vi "SVT Start Swept Sine (DAQmx).vi"(8 "error in (no error)":errorcluster, 11 "swept sine task in":T1={"source settings"={"AO task name"="", "source"=[]}, "stimulus settings"={"stimulus task name"="", "stimulus"=[]}, "response(s) settings"={"response task name"="", "response"=[]}, "measurement settings"={"AI sampling frequency"=51200.0, "AO sampling frequency"=1024.0, "AI block size"=1024, "AO block Size"=1024, "block duration [ms]"=0.0, "number of AI channels"=0, "device propagation delay [samples]"=0.0, "total propagation time [samples]"=0.0, "DUT propagation time [ms]"=0.0}, "linlog"=enum."linear", "repeat"=enum."off", "frequency list"=[1.0], "amplitude list"=[1.0], "settling time"={"settle time"=0.015599999576807022, "settle cycles"=5}, "integration time"={"integration time"=0.015599999576807022, "integration cycles"=5}, "frequencies indices"={"AI freq index"=0, "AO freq index"=5}, "read marks"={"write index"=0, "read index"=0, "freq start index"=0, "freq stop index"=0, "# extracted"=0, "buffer type"=enum."Invalid buffer", "read/write indices"=[], "AO index"=0, "AI index"=0, "settled"=FALSE, "integration done"=FALSE}, "harmonic settings"={"maximum THD harmonic"=5, "harmonic mapping"=[1], "units"={"THD unit"=enum."%", "nth harmonic unit"=enum."%", "SINAD unit"=enum."dB", "THD+N unit"=enum."dB"}}, "auto resolution settings"={"auto max step"=512, "slow threshold db"=6.0, "fast threshold db"=1.0}, "auto level settings"={"auto level enable"=FALSE, "auto level channel"=6, "ideal ref"=1.0, "max level"=10.0, "ref upper deviation db"=3.0, "ref lower deviation db"=-3.0}, "offset"=1.0, "ramping rate"=0.0, "phase"=1.0, "initialize"=FALSE} {"phase" format="%.2f"; "response(s) settings"."response"."channel info"."pregain" format="%.2f"; "response(s) settings"."response"."channel info"."weighting filter" items=["Linear", "A-weighting", "B-weighting", "C-weighting", "ITU-R 468-4", "Dolby", "CCITT", "C-message", "Wb", "Wc", "Wd", "We", "Wf", "Wh", "Wj", "Wk", "Wm", "AES17 20 kHz lowpass", "AES17 40 kHz lowpass", "AES17 20 kHz highpass", "AES17 40 kHz highpass"]; "response(s) settings"."response"."channel info"."dB reference" format="%^.1e"; "response(s) settings"."response"."channel info"."engineering units" items=["custom..."=0, "V"=1, "A"=21, "C"=30, "pC"=31, "s"=32, "-"=29, "Pa"=2, "N"=20, "g"=3, "m/s^2"=4, "m/s"=5, "m"=6, "mm/s"=12, "mm"=13, "micron/s"=14, "micron"=15, "in/s^2"=7, "in/s"=8, "in"=9, "mil/s"=10, "mil"=11, "rad/s^2"=16, "rad/s"=17, "rad"=18, "deg/s^2"=26, "deg/s"=27, "deg"=28, "RPM"=22, "cycle/s^2"=23, "Hz"=24, "cycle"=25, "strain"=19]; "response(s) settings"."response"."channel info"."sensor sensitivity" format="%#_5f"; "stimulus settings"."stimulus"."channel info"."pregain" format="%.2f"; "stimulus settings"."stimulus"."channel info"."weighting filter" items=["Linear", "A-weighting", "B-weighting", "C-weighting", "ITU-R 468-4", "Dolby", "CCITT", "C-message", "Wb", "Wc", "Wd", "We", "Wf", "Wh", "Wj", "Wk", "Wm", "AES17 20 kHz lowpass", "AES17 40 kHz lowpass", "AES17 20 kHz highpass", "AES17 40 kHz highpass"]; "stimulus settings"."stimulus"."channel info"."dB reference" format="%^.1e"; "stimulus settings"."stimulus"."channel info"."engineering units" items=["custom..."=0, "V"=1, "A"=21, "C"=30, "pC"=31, "s"=32, "-"=29, "Pa"=2, "N"=20, "g"=3, "m/s^2"=4, "m/s"=5, "m"=6, "mm/s"=12, "mm"=13, "micron/s"=14, "micron"=15, "in/s^2"=7, "in/s"=8, "in"=9, "mil/s"=10, "mil"=11, "rad/s^2"=16, "rad/s"=17, "rad"=18, "deg/s^2"=26, "deg/s"=27, "deg"=28, "RPM"=22, "cycle/s^2"=23, "Hz"=24, "cycle"=25, "strain"=19]; "stimulus settings"."stimulus"."channel info"."sensor sensitivity" format="%#_5f"; "ramping rate" format="%.4f"; "offset" format="%.2f"; "auto level settings"."ref lower deviation db" format="%.4f"; "auto level settings"."ref upper deviation db" format="%.4f"; "auto level settings"."max level" format="%.4f"; "auto level settings"."ideal ref" format="%.4f"; "auto resolution settings"."fast threshold db" format="%.4f"; "auto resolution settings"."slow threshold db" format="%.4f"; "harmonic settings"."maximum THD harmonic" max=10 step=1; "integration time"."integration time" format="%.2p"; "settling time"."settle time" format="%.2p"; "amplitude list" format="%.2f"; "frequency list" format="%.2f"; "measurement settings"."DUT propagation time [ms]" format="%.2f"; "measurement settings"."AO sampling frequency" format="%.2f"; "measurement settings"."AI sampling frequency" format="%.2f"}) -> (0 "error out":errorcluster, 3 "swept sine task out":T1={"source settings"={"AO task name"="", "source"=[]}, "stimulus settings"={"stimulus task name"="", "stimulus"=[]}, "response(s) settings"={"response task name"="", "response"=[]}, "measurement settings"={"AI sampling frequency"=51200.0, "AO sampling frequency"=1024.0, "AI block size"=1024, "AO block Size"=1024, "block duration [ms]"=0.0, "number of AI channels"=0, "device propagation delay [samples]"=0.0, "total propagation time [samples]"=0.0, "DUT propagation time [ms]"=0.0}, "linlog"=enum."linear", "repeat"=enum."off", "frequency list"=[1.0], "amplitude list"=[1.0], "settling time"={"settle time"=0.015599999576807022, "settle cycles"=5}, "integration time"={"integration time"=0.015599999576807022, "integration cycles"=5}, "frequencies indices"={"AI freq index"=0, "AO freq index"=5}, "read marks"={"write index"=0, "read index"=0, "freq start index"=0, "freq stop index"=0, "# extracted"=0, "buffer type"=enum."Invalid buffer", "read/write indices"=[], "AO index"=0, "AI index"=0, "settled"=FALSE, "integration done"=FALSE}, "harmonic settings"={"maximum THD harmonic"=5, "harmonic mapping"=[1], "units"={"THD unit"=enum."%", "nth harmonic unit"=enum."%", "SINAD unit"=enum."dB", "THD+N unit"=enum."dB"}}, "auto resolution settings"={"auto max step"=512, "slow threshold db"=6.0, "fast threshold db"=1.0}, "auto level settings"={"auto level enable"=FALSE, "auto level channel"=6, "ideal ref"=1.0, "max level"=10.0, "ref upper deviation db"=3.0, "ref lower deviation db"=-3.0}, "offset"=1.0, "ramping rate"=0.0, "phase"=1.0, "initialize"=FALSE} {"phase" format="%.2f"; "response(s) settings"."response"."channel info"."pregain" format="%.2f"; "response(s) settings"."response"."channel info"."weighting filter" items=["Linear", "A-weighting", "B-weighting", "C-weighting", "ITU-R 468-4", "Dolby", "CCITT", "C-message", "Wb", "Wc", "Wd", "We", "Wf", "Wh", "Wj", "Wk", "Wm", "AES17 20 kHz lowpass", "AES17 40 kHz lowpass", "AES17 20 kHz highpass", "AES17 40 kHz highpass"]; "response(s) settings"."response"."channel info"."dB reference" format="%^.1e"; "response(s) settings"."response"."channel info"."engineering units" items=["custom..."=0, "V"=1, "A"=21, "C"=30, "pC"=31, "s"=32, "-"=29, "Pa"=2, "N"=20, "g"=3, "m/s^2"=4, "m/s"=5, "m"=6, "mm/s"=12, "mm"=13, "micron/s"=14, "micron"=15, "in/s^2"=7, "in/s"=8, "in"=9, "mil/s"=10, "mil"=11, "rad/s^2"=16, "rad/s"=17, "rad"=18, "deg/s^2"=26, "deg/s"=27, "deg"=28, "RPM"=22, "cycle/s^2"=23, "Hz"=24, "cycle"=25, "strain"=19]; "response(s) settings"."response"."channel info"."sensor sensitivity" format="%#_5f"; "stimulus settings"."stimulus"."channel info"."pregain" format="%.2f"; "stimulus settings"."stimulus"."channel info"."weighting filter" items=["Linear", "A-weighting", "B-weighting", "C-weighting", "ITU-R 468-4", "Dolby", "CCITT", "C-message", "Wb", "Wc", "Wd", "We", "Wf", "Wh", "Wj", "Wk", "Wm", "AES17 20 kHz lowpass", "AES17 40 kHz lowpass", "AES17 20 kHz highpass", "AES17 40 kHz highpass"]; "stimulus settings"."stimulus"."channel info"."dB reference" format="%^.1e"; "stimulus settings"."stimulus"."channel info"."engineering units" items=["custom..."=0, "V"=1, "A"=21, "C"=30, "pC"=31, "s"=32, "-"=29, "Pa"=2, "N"=20, "g"=3, "m/s^2"=4, "m/s"=5, "m"=6, "mm/s"=12, "mm"=13, "micron/s"=14, "micron"=15, "in/s^2"=7, "in/s"=8, "in"=9, "mil/s"=10, "mil"=11, "rad/s^2"=16, "rad/s"=17, "rad"=18, "deg/s^2"=26, "deg/s"=27, "deg"=28, "RPM"=22, "cycle/s^2"=23, "Hz"=24, "cycle"=25, "strain"=19]; "stimulus settings"."stimulus"."channel info"."sensor sensitivity" format="%#_5f"; "ramping rate" format="%.4f"; "offset" format="%.2f"; "auto level settings"."ref lower deviation db" format="%.4f"; "auto level settings"."ref upper deviation db" format="%.4f"; "auto level settings"."max level" format="%.4f"; "auto level settings"."ideal ref" format="%.4f"; "auto resolution settings"."fast threshold db" format="%.4f"; "auto resolution settings"."slow threshold db" format="%.4f"; "harmonic settings"."maximum THD harmonic" max=10 step=1; "integration time"."integration time" format="%.2p"; "settling time"."settle time" format="%.2p"; "amplitude list" format="%.2f"; "frequency list" format="%.2f"; "measurement settings"."DUT propagation time [ms]" format="%.2f"; "measurement settings"."AO sampling frequency" format="%.2f"; "measurement settings"."AI sampling frequency" format="%.2f"})   [LabVIEW 2017, in "SoundVib_SweptSine.lvlib"]
doc: "Starts the swept-sine measurement."
uses:
  <vilib>/addons/Sound and Vibration/svt_Swept Sine/SoundVib_SweptSine.lvlib
  <vilib>/addons/Sound and Vibration/svt_Swept Sine/subVIs/sv_Swept Sine Task.ctl
  <vilib>/addons/_NISVFA/_Shared subVIs/Controls/svc_Channel Info.ctl
  <vilib>/addons/_NISVFA/_Shared subVIs/Controls/svc_Engineering Units Text Ring.ctl
  <vilib>/addons/_NISVFA/_Shared subVIs/Controls/svc_Weighting Filter Text Ring.ctl
  <vilib>/DAQmx/write.llb/DAQmx Write (Analog 1D DBL 1Chan NSamp).vi
  <vilib>/DAQmx/miscellaneous.llb/DAQmx Fill In Error Info.vi
  <vilib>/DAQmx/configure/trigger.llb/DAQmx Start Trigger (Digital Edge).vi
  <resource>/objmgr/daqmx.rc
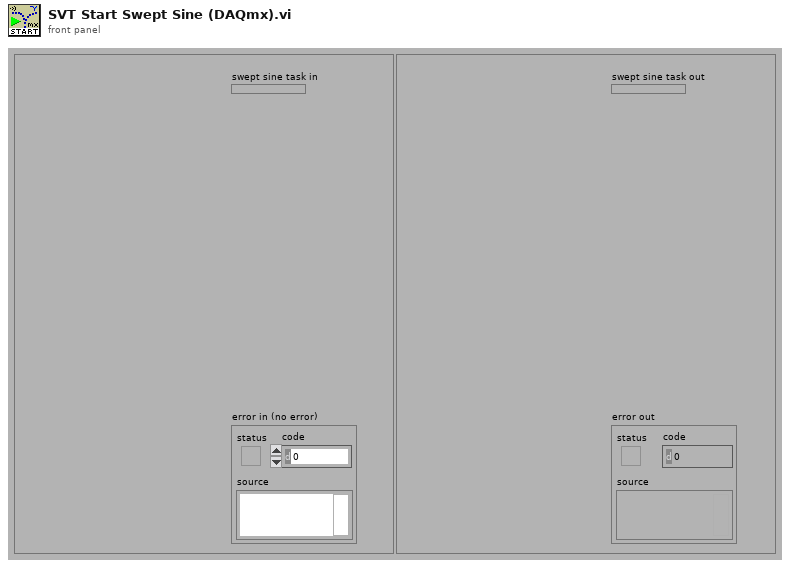
[diagram p1: front panel]
types:
  T1 = typedef "SoundVib_SweptSine.lvlib/sv_Swept Sine Task.ctl" = cluster{"source settings":cluster{"AO task name":refnum<k21>, "source":cluster{"AO physical channel":tag}[]}, "stimulus settings":cluster{"stimulus task name":refnum<k21>, "stimulus":cluster{"stimulus physical channel":tag, "channel info":T2}[]}, "response(s) settings":cluster{"response task name":refnum<k21>, "response":cluster{"response physical channel":tag, "channel info":T2}[]}, "measurement settings":cluster{"AI sampling frequency":dbl, "AO sampling frequency":dbl, "AI block size":i32, "AO block Size":i32, "block duration [ms]":dbl, "number of AI channels":i32, "device propagation delay [samples]":dbl, "total propagation time [samples]":dbl, "DUT propagation time [ms]":dbl}, "linlog":enum16{"linear", "log"}, "repeat":enum16{"off", "on"}, "frequency list":dbl[], "amplitude list":dbl[], "settling time":cluster{"settle time":dbl, "settle cycles":i32}, "integration time":cluster{"integration time":dbl, "integration cycles":i32}, "frequencies indices":cluster{"AI freq index":i32, "AO freq index":i32}, "read marks":cluster{"write index":u32, "read index":u32, "freq start index":u32, "freq stop index":u32, "# extracted":u32, "buffer type":enum16{"Invalid buffer", "Intermediate buffer", "Final buffer"}, "read/write indices":cluster{"settle time index":u32, "integration time index":u32}[], "AO index":i32, "AI index":i32, "settled":bool, "integration done":bool}, "harmonic settings":cluster{"maximum THD harmonic":u32, "harmonic mapping":u32[], "units":cluster{"THD unit":enum16{"dB", "%"}, "nth harmonic unit":enum16{"dB", "%"}, "SINAD unit":enum16{"dB", "%"}, "THD+N unit":enum16{"dB", "%"}}}, "auto resolution settings":cluster{"auto max step":i32, "slow threshold db":dbl, "fast threshold db":dbl}, "auto level settings":cluster{"auto level enable":bool, "auto level channel":u8, "ideal ref":sgl, "max level":sgl, "ref upper deviation db":sgl, "ref lower deviation db":sgl}, "offset":dbl, "ramping rate":dbl, "phase":dbl, "initialize":bool}
  T2 = typedef "svc_Channel Info.ctl" = cluster{"sensor sensitivity":dbl, "engineering units":T3, "dB reference":dbl, "custom label":string, "weighting filter":T4, "pregain":dbl}
  T3 = typedef "svc_Engineering Units Text Ring.ctl" = u16
  T4 = typedef "svc_Weighting Filter Text Ring.ctl" = u16
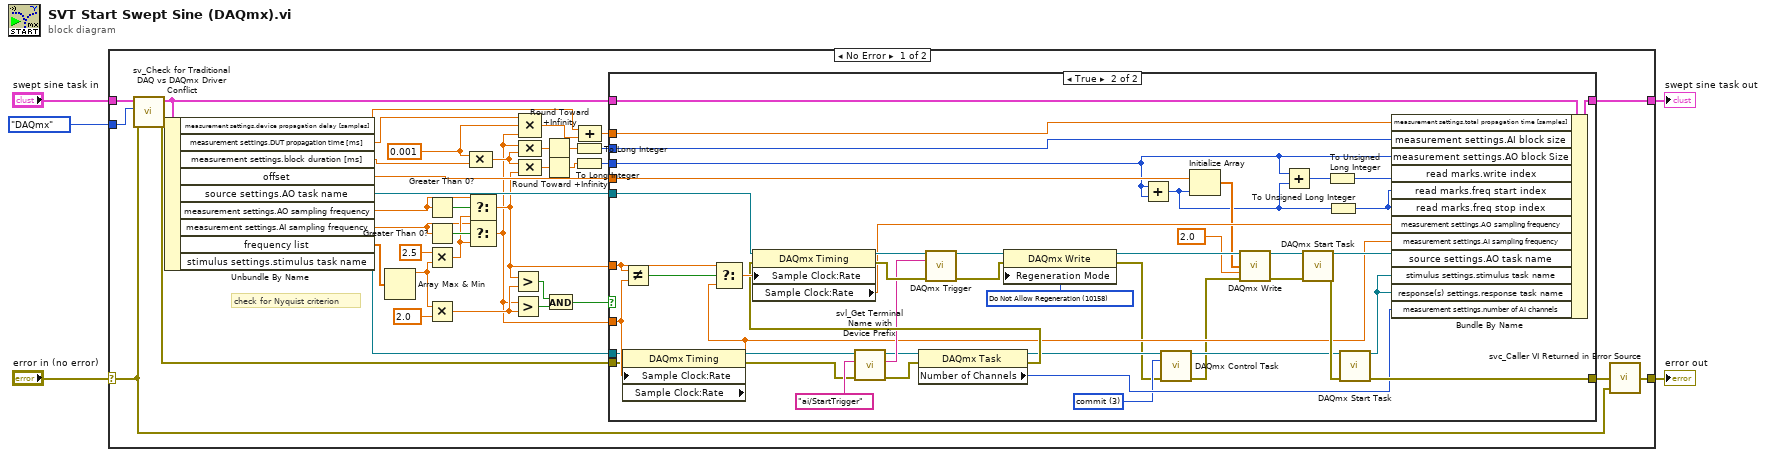
[diagram p0: block diagram]
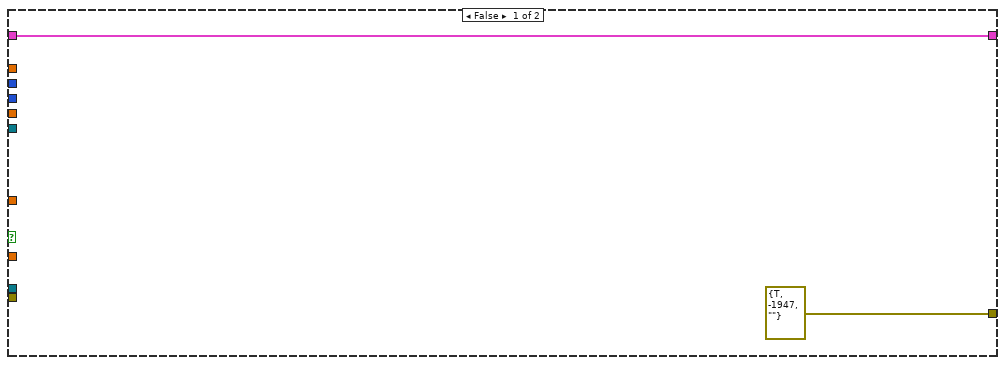
[diagram p2: hidden frame]
diagram:
  n1 = case shown="No Error" "error in (no error)" {
    selector: "error in (no error)" -> [w36 w93]
    tunnel: [w40 w93] -> w5
    tunnel: [w43 w94] -> w4
    tunnel: "swept sine task in" -> [w39 w94]
    tunnel: enum16{"DAQmx", "Traditional DAQ"}."DAQmx" ("device driver") -> [w24 _]
    frame No Error {
      w6 = 0.001 ("x")
      # "check for Nyquist criterion"
      n2 = call <vilib>:"sv_Check for Traditional DAQ vs DAQmx Driver Conflict.vi"("error in (no error)"=w36, "device driver"=w24, "swept sine task"=w39) -> ("error out"=w38:errorcluster, "dup swept sine task"=w12:T1)  [unwired: 7 in]
      n3 = Unbundle By Name(w12) -> ("measurement settings.device propagation delay [samples]"=w10:dbl, "measurement settings.DUT propagation time [ms]"=w7:dbl, "measurement settings.block duration [ms]"=w23:dbl, "offset"=w37:dbl, "source settings.AO task name"=w44:refnum<k21>, "measurement settings.AO sampling frequency"=w26:dbl, "measurement settings.AI sampling frequency"=w25:dbl, "frequency list"=w42:dbl[], "stimulus settings.stimulus task name"=w14:refnum<k21>)
      n4 = Array Max & Min(array=w42) -> (max value=w22:dbl)  [unwired: 3 out]
      n5 = Greater Than 0?(x=w26) -> (x > 0?=w33:bool)
      n6 = Greater Than 0?(x=w25) -> (x > 0?=w34:bool)
      n7 = Multiply(x=2.5 ("y"), y=w22) -> (x*y=w32:dbl)
      n8 = Multiply(x=w22, y=2.0) -> (x*y=w18:dbl)
      n9 = Select(t=w26, s=w33, f=w32) -> (s? t:f=w16:dbl)
      n10 = Select(t=w25, s=w34, f=w32) -> (s? t:f=w9:dbl)
      n11 = Compound Arithmetic op=MULTIPLY(w6, w23) -> (w27:dbl)
      n12 = Greater?(x=w16, y=w18) -> (0:w19:bool)
      n13 = Greater?(x=w9, y=w18) -> (0:w20:bool)
      n14 = Compound Arithmetic op=MULTIPLY(w7, w6, w9) -> (w8:dbl)
      n15 = Compound Arithmetic op=MULTIPLY(w9, w27) -> (w28:dbl)
      n16 = Compound Arithmetic op=MULTIPLY(w27, w16) -> (w30:dbl)
      n17 = Round Toward +Infinity(x=w28) -> (ceil(x): smallest int >= x=w29:dbl)
      n18 = Round Toward +Infinity(x=w30) -> (ceil(x): smallest int >= x=w31:dbl)
      n19 = And(x=w19, y=w20) -> (x .and. y?=w17:bool)
      n20 = To Long Integer(number=w29) -> (32bit integer=w13:i32)
      n21 = To Long Integer(number=w31) -> (32bit integer=w15:i32)
      n22 = Compound Arithmetic op=ADD(w10, w8) -> (w11:dbl)
      n23 = case shown="True" w17 {
        tunnel: w44 -> [_ w67]
        tunnel: w16 -> [_ w47]
        tunnel: w9 -> [_ w68]
        tunnel: [errorcluster {"status"=TRUE, "code"=-1947, "source"=""} ("error in (no error)") w81] -> w41
        tunnel: w12 -> [w46 w78]
        tunnel: [w46 w83] -> w43
        tunnel: w38 -> [_ w63]
        tunnel: w14 -> [_ w66]
        tunnel: w37 -> [_ w77]
        tunnel: w15 -> [_ w58]
        tunnel: w13 -> [_ w59]
        tunnel: w11 -> [_ w60]
        frame False {
        }
        frame True {
          w52 = 3 items=["verify"=2, "reserve"=4, "commit"=3, "unreserve"=5, "abort"=6] ("action")
          w88 = 10158 items=["Allow Regeneration"=10097, "Do Not Allow Regeneration"=10158] ("RegenMode")
          n24 = Not Equal?(x=w47, y=w68) -> (x != y?=w75:bool)
          n25 = property class="DAQmx Timing"(reference=w66, error in=w63, "Sample Clock:Rate"=w68) -> (reference out=w71:refnum<k21>, error out=w74:errorcluster, "Sample Clock:Rate"=w55:dbl)
          n26 = Select(t=w47, s=w75, f=w55) -> (s? t:f=w65:dbl)
          n27 = call <vilib>:"svl_Get Terminal Name with Device Prefix.vi"("error in (no error)"=w74, "local terminal name"="ai/StartTrigger", "task/channels in"=w71) -> ("error out"=w48:errorcluster, "terminal name with device prefix"=w61:tag, "task out"=w49:refnum<k21>)  [unwired: 6 in]
          n28 = property class="DAQmx Task"(reference=w49, error in=w48) -> (reference out=w54:refnum<k21>, error out=w64:errorcluster, "Number of Channels"=w62:u32)
          n29 = property class="DAQmx Timing"(reference=w67, error in=w64, "Sample Clock:Rate"=w65) -> (reference out=w73:refnum<k21>, error out=w72:errorcluster, "Sample Clock:Rate"=w69:dbl)
          n30 = call-poly <vilib>:"DAQmx Trigger.vi"("task/channels in"=w73, "source"=w61, "error in"=w72) -> ("task out"=w91:refnum<k21>, "error out"=w90:errorcluster)  [unwired: 11 in]
          n31 = property class="DAQmx Write"(reference=w91, error in=w90, "Regeneration Mode"=w88) -> (reference out=w89:refnum<k21>, error out=w51:errorcluster)
          n32 = Add(x=w58, y=w58) -> (x+y=w56:i32)
          n33 = call <vilib>:"DAQmx Control Task.vi"("task/channels in"=w54, "action"=w52, "error in"=w51) -> ("task out"=w53:refnum<k21>, "error out"=w50:errorcluster)  [unwired: 11 in]
          n34 = Initialize Array(w77, w56) -> (w57:dbl[])
          n35 = call-poly <vilib>:"DAQmx Write.vi"("task/channels in"=w89, "data"=w57, "timeout"=2.0 ("Wirite Timeout"), "error in"=w50) -> ("task out"=w92:refnum<k21>, "error out"=w70:errorcluster)  [unwired: 9 in, 1 out]
          n36 = Add(x=w58, y=w56) -> (x+y=w84:i32)
          n37 = call <vilib>:"DAQmx Start Task.vi"("task/channels in"=w92, "error in"=w70) -> ("task out"=w80:refnum<k21>, "error out"=w82:errorcluster)  [unwired: 12 in]
          n38 = To Unsigned Long Integer(number=w84) -> (unsigned 32bit integer=w85:u32)
          n39 = To Unsigned Long Integer(number=w56) -> (unsigned 32bit integer=w86:u32)
          n40 = call <vilib>:"DAQmx Start Task.vi"("task/channels in"=w53, "error in"=w82) -> ("task out"=w79:refnum<k21>, "error out"=w81:errorcluster)  [unwired: 12 in]
          n41 = Bundle By Name(cluster=w78, "measurement settings.total propagation time [samples]"=w60, "measurement settings.AI block size"=w59, "measurement settings.AO block Size"=w58, "read marks.write index"=w85, "read marks.freq start index"=w86, "read marks.freq stop index"=w86, "measurement settings.AO sampling frequency"=w69, "measurement settings.AI sampling frequency"=w55, "source settings.AO task name"=w80, "stimulus settings.stimulus task name"=w79, "response(s) settings.response task name"=w79, "measurement settings.number of AI channels"=w62) -> (w83:T1)
        }
      }
      n42 = call <vilib>:"svc_Caller VI Returned in Error Source.vi"("warning input to caller"=w36, "error in (no error)"=w41) -> ("error out"=w40:errorcluster)  [unwired: 3 in]
    }
    frame Error {
    }
  }
  "error out" <- w5
  "swept sine task out" <- w4
